vi "Merge_Grouped_Tracks_Values-1.vi"(3 "[IN] Testing Frame":u32 min=24 max=58, 4 "[IN] Tracks group":i32 min=0 max=258, 5 "[IN] Grouped Tracks":T2(array[cluster])) -> (1 "[OUT] Grouped Tracks Values":T1)   [LabVIEW 2013]
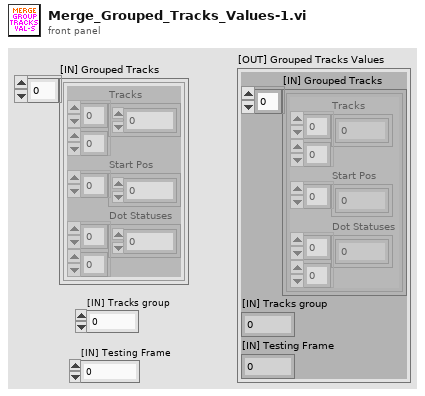
[diagram p1: front panel]
types:
  T1 = cluster{"[IN] Grouped Tracks":cluster{"Tracks":dbl[][], "Start Pos":i32[], "Dot Statuses":i16[][]}[], "[IN] Tracks group":i32, "[IN] Testing Frame ":u32}
  T2 = cluster{"Tracks":dbl[][], "Start Pos":i32[], "Dot Statuses":i16[][]}[]
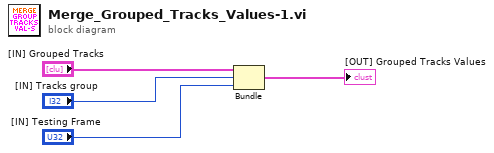
[diagram p0: block diagram]
diagram:
  n1 = Bundle("[IN] Grouped Tracks"="[IN] Grouped Tracks", "[IN] Tracks group"="[IN] Tracks group", "[IN] Testing Frame"="[IN] Testing Frame") -> (→"[OUT] Grouped Tracks Values":T1)  [unwired: 1 in]
